vi "AlliGator Add Decay Shift to Plot.vi"(9 "Decay Shift":dbl, 10 "Time Stamp":dbl, 11 "Decay Shift Plot in":T1) -> (3 "Decay Shift Plot out":T1)   [LabVIEW 2021, in "AlliGator Decay Processing.lvlib"]
doc: "Adds timestamp and decay shift to internal variables when computing a new decay."
uses:
  AlliGator Decay Processing.lvlib
panel:
  # "see the AlliGator License on the block diagram (Ctrl+E or Window:Show Block Diagram)"
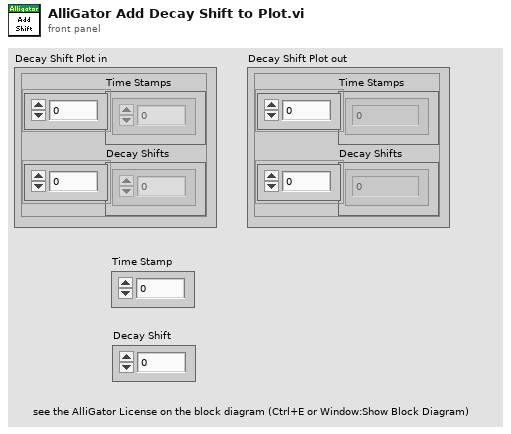
[diagram p1: front panel]
types:
  T1 = cluster{"Time Stamps":dbl[], "Decay Shifts":dbl[]}
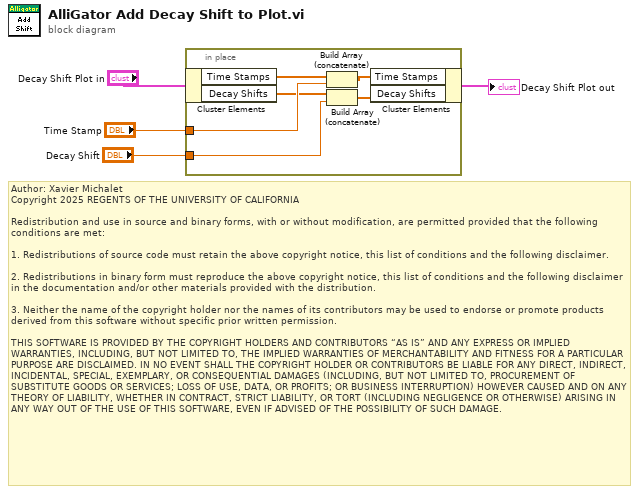
[diagram p0: block diagram]
diagram:
  # "Author: Xavier Michalet\nCopyright 2025 REGENTS OF THE UNIVERSITY OF CALIFORNIA\n\nRedistribution and use in source and binary forms, with or without modification, are permitted provided that the following conditions are met:\n\n1. Redistributions of source code must retain the above copyright notice, this list of conditions and the following disclaimer.\n\n2. Redistributions in binary form must reproduce the above copyright notice, this list of conditions and the following disclaimer in the documentation and/or other materials provided with the distribution.\n\n3. Neither the name of the copyright holder nor the names of its contributors may be used to endorse or promote products derived from this software without specific prior written permission.\n\nTHIS SOFTWARE IS PROVIDED BY THE COPYRIGHT HOLDERS AND CONTRIBUTORS “AS IS” AND ANY EXPRESS OR IMPLIED WARRANTIES, INCLUDING, BUT NOT LIMITED TO, THE IMPLIED WARRANTIES OF MERCHANTABILITY AND FITNESS FOR A PARTICULAR PURPOSE ARE DISCLAIMED. IN NO EVENT SHALL THE COPYRIGHT HOLDER OR CONTRIBUTORS BE LIABLE FOR ANY DIRECT, INDIRECT, INCIDENTAL, SPECIAL, EXEMPLARY, OR CONSEQUENTIAL DAMAGES (INCLUDING, BUT NOT LIMITED TO, PROCUREMENT OF SUBSTITUTE GOODS OR SERVICES; LOSS OF USE, DATA, OR PROFITS; OR BUSINESS INTERRUPTION) HOWEVER CAUSED AND ON ANY THEORY OF LIABILITY, WHETHER IN CONTRACT, STRICT LIABILITY, OR TORT (INCLUDING NEGLIGENCE OR OTHERWISE) ARISING IN ANY WAY OUT OF THE USE OF THIS SOFTWARE, EVEN IF ADVISED OF THE POSSIBILITY OF SUCH DAMAGE."
  n1 = in-place {
    in-place-border: "Time Stamp" -> [w10]
    in-place-border: "Decay Shift" -> [w9]
    n2 = in-place-cluster #1("Decay Shift Plot in") -> ("Time Stamps"=w8:dbl[], "Decay Shifts"=w6:dbl[])
    n3 = Build Array (concatenate)(w8, w10) -> (w7:dbl[])
    n4 = Build Array (concatenate)(w6, w9) -> (w5:dbl[])
    n5 = in-place-cluster #1("Time Stamps"=w7, "Decay Shifts"=w5) -> (→"Decay Shift Plot out":T1)
  }
